vi "Set Units.vi"(8 "error in (no error)":errorcluster, 9 "Units":string, 10 "Channel":T1, 11 "EPU452 in":refnum<class "EPU452.lvclass">) -> (0 "error out":errorcluster, 2 "Response":string, 3 "EPU452 out":refnum<class "EPU452.lvclass">)   [LabVIEW 2018, in "EPU452.lvclass"]
uses:
  EPU452.lvclass
  Controls/Channels.ctl
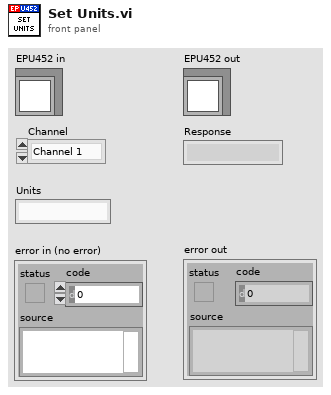
[diagram p1: front panel]
types:
  T1 = typedef "EPU452.lvclass/Channels.ctl" = enum16{"Channel 1", "Channel 2", "Channel 3", "Channel 4"}
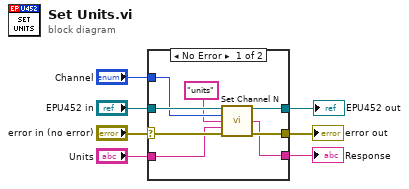
[diagram p0: block diagram]
diagram:
  n1 = case shown="No Error" "error in (no error)" {
    selector: "error in (no error)" -> [w12 w17]
    tunnel: [w9 w17] -> w6
    tunnel: [w10 w16] -> w4
    tunnel: "EPU452 in" -> [w15 w16]
    tunnel: "Channel" -> [w14 _]
    tunnel: "Units" -> [w11 _]
    tunnel: [w8 _] -> w1
    frame No Error {
      n2 = call "Set Channel N.vi"("EPU452 in"=w15, "Channel"=w14, "Function"="units", "Argument/s"=w11, "error in (no error)"=w12) -> ("EPU452 out"=w10:refnum<class "EPU452.lvclass">, "Response"=w8:string, "error out"=w9:errorcluster)  [unwired: 8 in]
    }
    frame Error {
    }
  }
  "error out" <- w6
  "EPU452 out" <- w4
  "Response" <- w1
